vi "Login.vi"() -> ()   [LabVIEW 2018]
doc: "SubVI criada para realizar login de usuários"
uses:
  controls/Table.ctl
  controls/DataIn.ctl
  MatchDataClasses/MatchData/MatchData.lvclass
  controls/Tabuleiro.ctl
  controls/GameOption.ctl
  controls/Login - States.ctl
  controls/LoginStatus.ctl
  <vilib>/Utility/file.llb/Read Delimited Spreadsheet (string).vi
  <vilib>/Utility/file.llb/Write Delimited Spreadsheet (string).vi
panel:
  out "DataOut":T1={"Quem Joga"="", "Tabuleiro"={"(0,0)"="", "(1,0)"="", "(0,1)"="", "(1,1)"="", "(2,0)"="", "(1,2)"="", "(2,2)"="", "(0,2)"="", "(2,1) "=""}, "GameOption"=enum."Multiplayer local", "Turno"=FALSE, "Player"="", "Player 1"="", "Player 2"="", "Dificuldade"=enum."Easy", "Table"=[], "Row"=0, "Aceitar Convite"=FALSE, "Inviter line"=0, "diretório"=path "", "Logout - panel close"=FALSE, "StartGame"=FALSE, "MatchData.lvclass"=refnum, "GameMode"=enum."Single Easy"}
  in  "logout":bool
  out "Table":T4
  in  "Login":bool
  in  "User Name":string
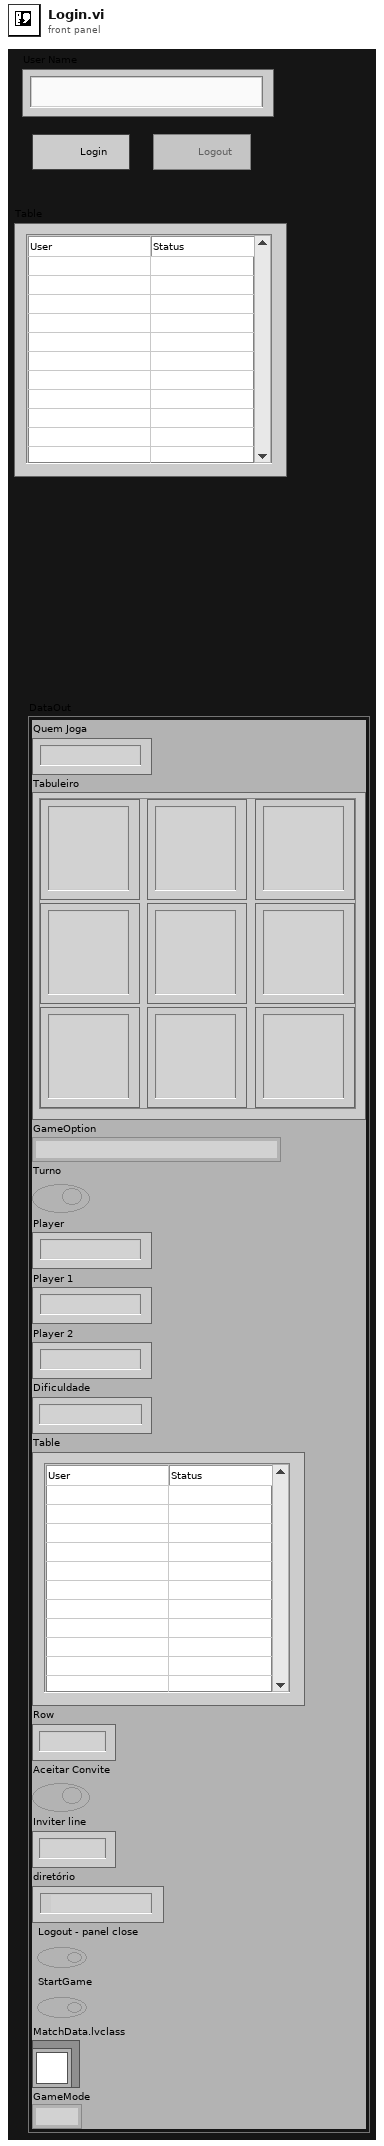
[diagram p1: front panel]
types:
  T1 = typedef "DataIn.ctl" = cluster{"Quem Joga":string, "Tabuleiro":T2, "GameOption":T3, "Turno":bool, "Player":string, "Player 1":string, "Player 2":string, "Dificuldade":enum16{"Easy", "Medium", "Hard"}, "Table":T4, "Row":u32, "Aceitar Convite":bool, "Inviter line":u32, "diretório":path, "Logout - panel close":bool, "StartGame":bool, "MatchData.lvclass":refnum<class "MatchData.lvclass">, "GameMode":enum16{"Single Easy", "Single Medium", "Single Hard", "Local", "Remote"}}
  T2 = typedef "Tabuleiro.ctl" = cluster{"(0,0)":string, "(1,0)":string, "(0,1)":string, "(1,1)":string, "(2,0)":string, "(1,2)":string, "(2,2)":string, "(0,2)":string, "(2,1) ":string}
  T3 = typedef "GameOption.ctl" = enum16{"Single Player", "Multiplayer local", "Multiplayer remoto", "Wait for Event", "Initialize", "Stop"}
  T4 = typedef "Table.ctl" = string[][]
  T5 = typedef "Login - States.ctl" = enum16{"Login - Initialize", "Login - Wait for Event", "Login", "Logout", "Table Refresh", "Invitation"}
  T6 = enum8{"Enabled", "Disabled", "Disabled and Grayed Out"}
  T7 = typedef "LoginStatus.ctl" = enum16{"File - Login", "File - Logout", "File - TableRefresh"}
  T8 = typedef "LVRowAndColumnTypeDef.ctl" = cluster{"Row":i32, "Column":i32}
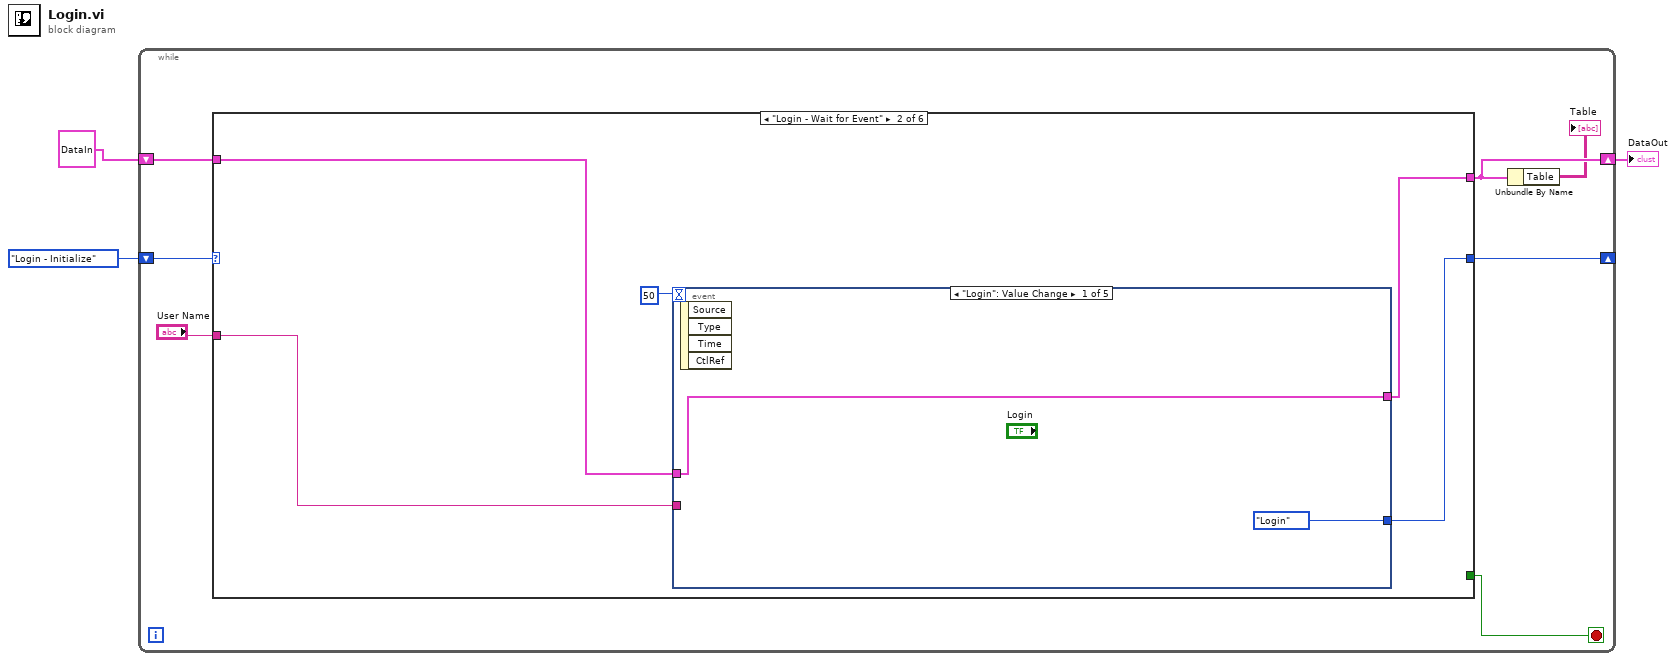
[diagram p0: block diagram]
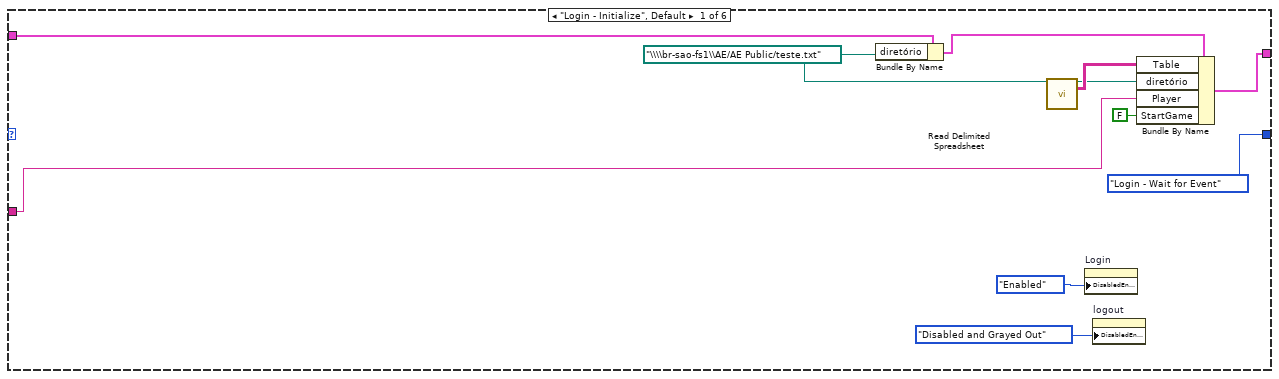
[diagram p2: hidden frame]
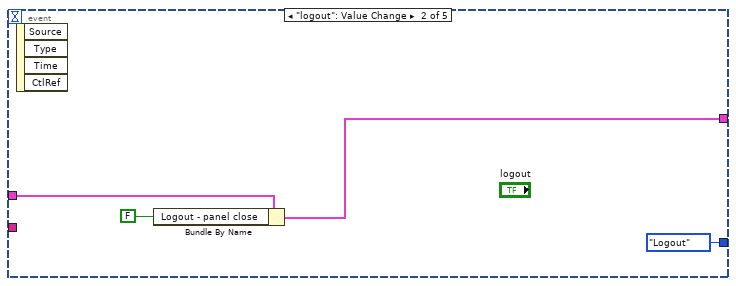
[diagram p3: hidden frame]
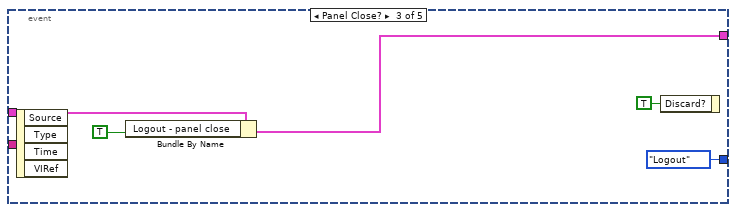
[diagram p4: hidden frame]
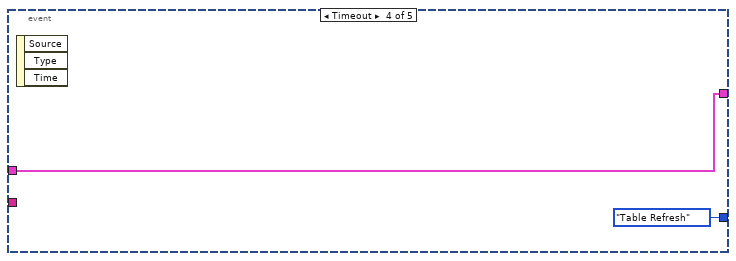
[diagram p5: hidden frame]
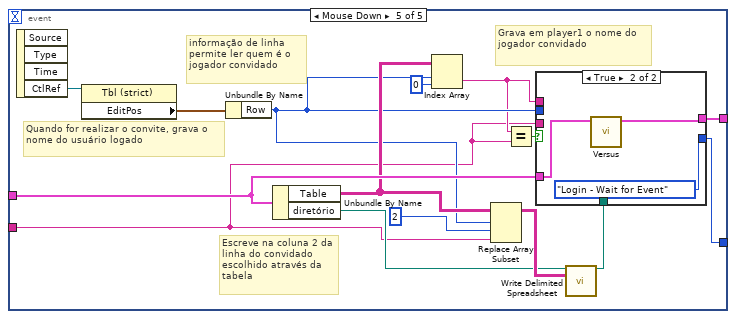
[diagram p6: hidden frame]
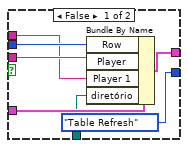
[diagram p7: hidden frame]
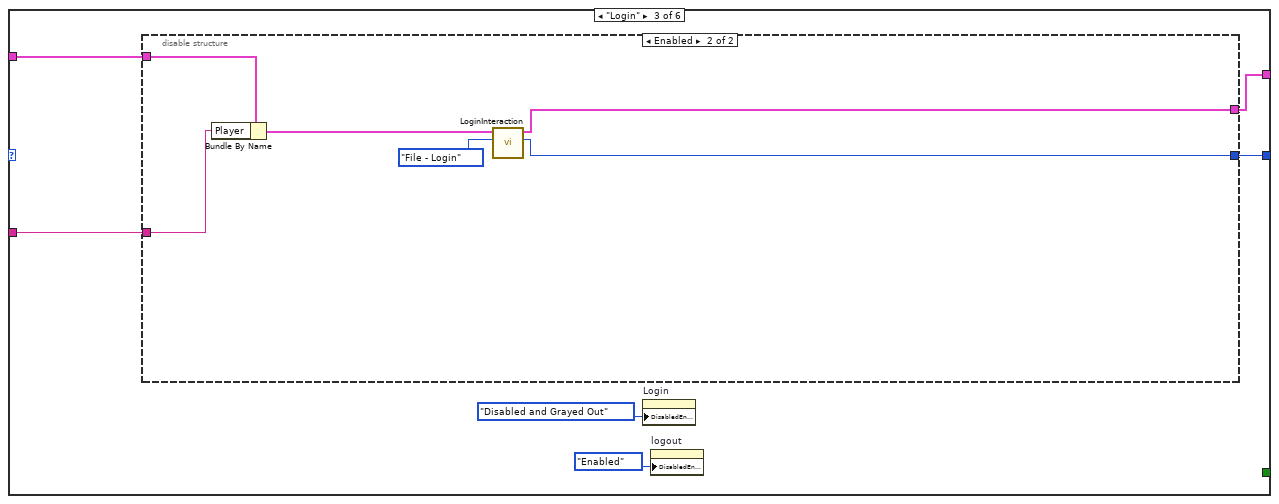
[diagram p8: hidden frame]
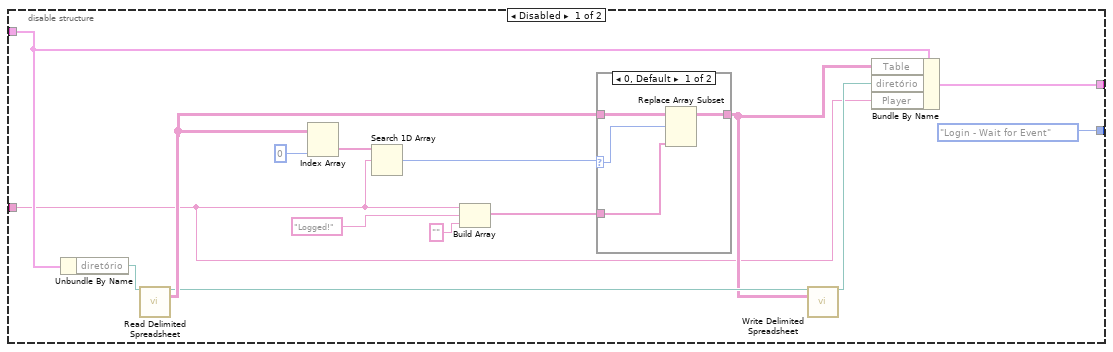
[diagram p9: hidden frame]
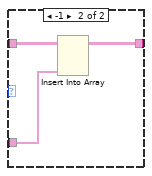
[diagram p10: hidden frame]
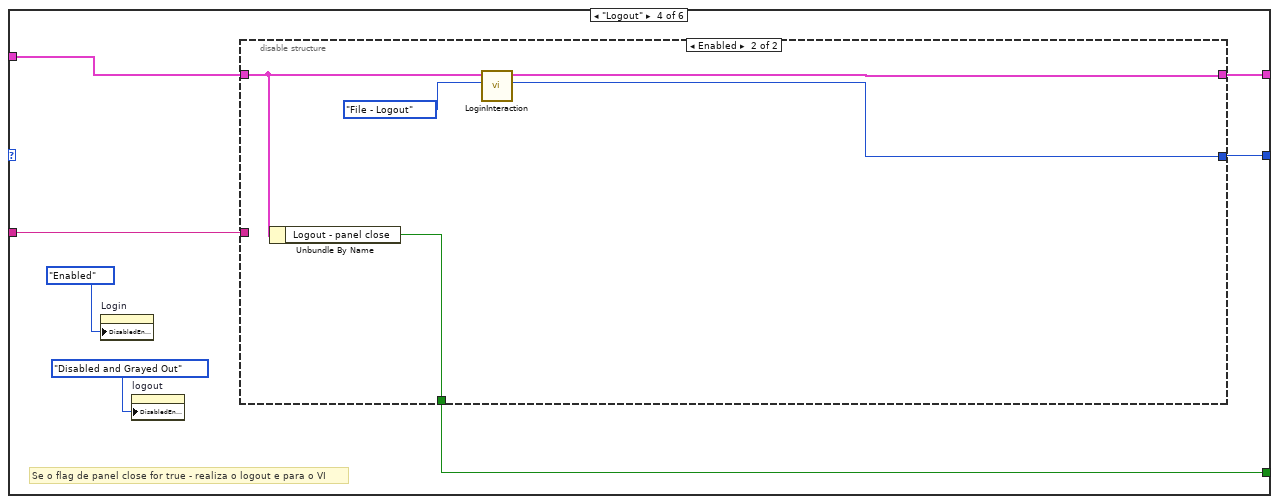
[diagram p11: hidden frame]
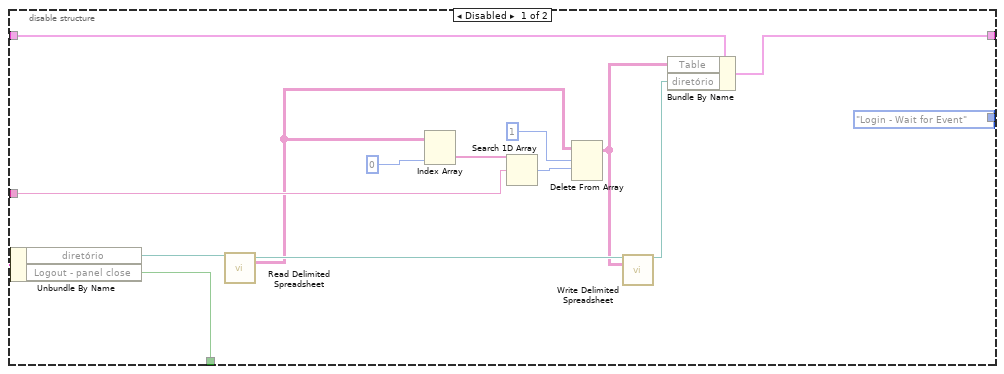
[diagram p12: hidden frame]
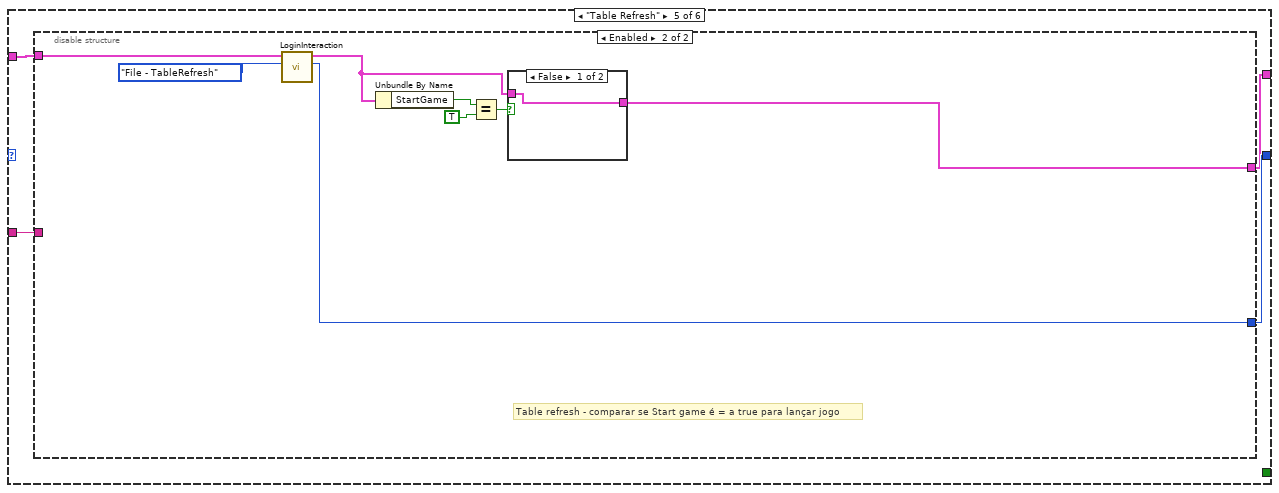
[diagram p13: hidden frame]
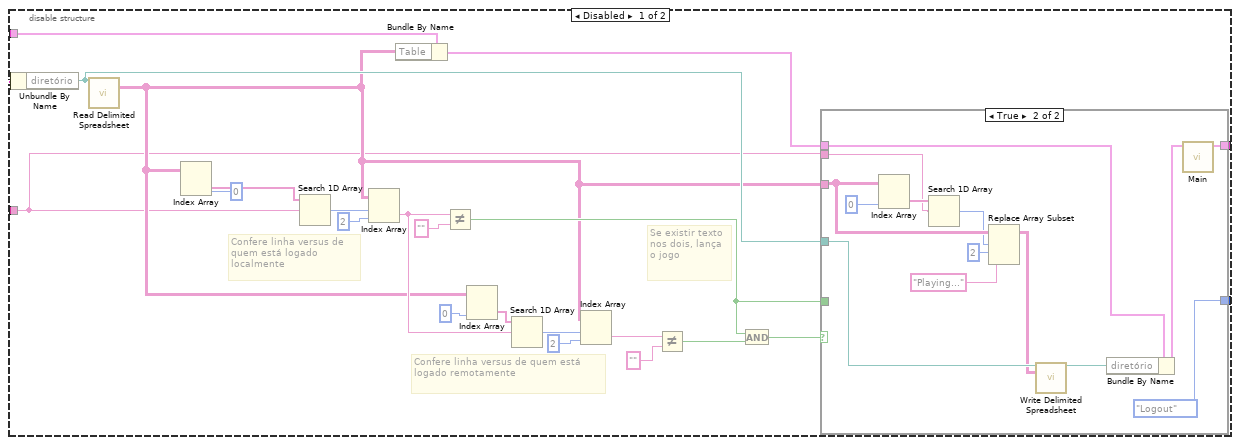
[diagram p14: hidden frame]
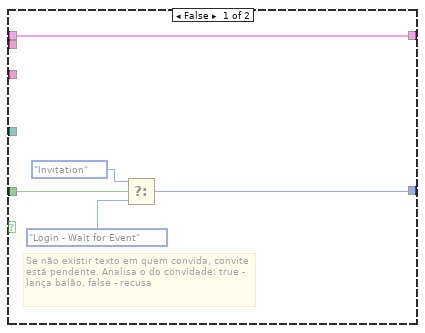
[diagram p15: hidden frame]
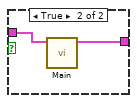
[diagram p16: hidden frame]
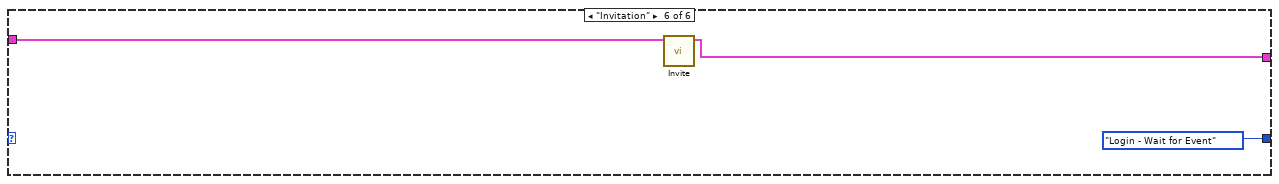
[diagram p17: hidden frame]
diagram:
  n1 = while {
    shift-right: [w9] -> _
    shift-left: Login_-_States."Login - Initialize" -> [w10]
    shift-right: [w5] -> w1
    shift-left: T1 {"Quem Joga"="", "Tabuleiro"={"(0,0)"="", "(1,0)"="", "(0,1)"="", "(1,1)"="", "(2,0)"="", "(1,2)"="", "(2,2)"="", "(0,2)"="", "(2,1) "=""}, "GameOption"=enum."Multiplayer local", "Turno"=FALSE, "Player"="", "Player 1"="", "Player 2"="", "Dificuldade"=enum."Easy", "Table"=[], "Row"=0, "Aceitar Convite"=FALSE, "Inviter line"=0, "diretório"=path "", "Logout - panel close"=FALSE, "StartGame"=FALSE, "MatchData.lvclass"=refnum, "GameMode"=enum."Single Easy"} ("DataIn") -> [w8]
    stop <- w6 stop-if-true
    n2 = case shown="\"Login - Wait for Event\"" w10 {
      tunnel: [Login_-_States."Login - Wait for Event" w26 w70 w104 w128 Login_-_States."Login - Wait for Event"] -> w9
      tunnel: w8 -> [w16 w23 w66 w99 w126 w182]
      tunnel: "User Name" -> [w12 w24 w65 w105 w125 _]
      tunnel: [_ _ _ w100 _ _] -> w6
      tunnel: [w18 w22 w67 w101 w127 w181] -> w5
      frame "Login - Initialize", Default {
        w14 = path "\\\\br-sao-fs1\\AE/AE Public/teste.txt" ("file path (use dialog)")
        n3 = Bundle By Name(cluster=w16, "diretório"=w14) -> (w15:T1)
        n4 = call-poly <vilib>:"Read Delimited Spreadsheet.vi"("file path (dialog if empty)"=w14) -> ("new file path (Not A Path if cancelled)"=w13:path, "all rows"=w17:string[][])  [unwired: 9 in, 4 out]
        n5 = property on="Login" class="Bool"("DisabledEnum"=T6."Enabled" ("Disabled")) -> ()  [unwired: 2 in, 2 out]
        n6 = property on="logout" class="Bool"("DisabledEnum"=T6."Disabled and Grayed Out" ("Disabled")) -> ()  [unwired: 2 in, 2 out]
        n7 = Bundle By Name(cluster=w15, "Table"=w17, "diretório"=w13, "Player"=w12, "StartGame"=FALSE) -> (w18:T1)
      }
      frame "Login - Wait for Event" {
        n8 = event shown="[0] \"Login\": Value Change" {
          selector: _ -> [_ _ _ _ _]
          dyn-events: _ -> [_ _ _ _ _]
          timeout: 50 -> [_ _ _ _ _]
          tunnel: [Login_-_States."Login" Login_-_States."Logout" Login_-_States."Logout" Login_-_States."Table Refresh" w40] -> w26
          tunnel: w23 -> [w27 w31 w35 w38 w51]
          tunnel: [w27 w30 w34 w38 w52] -> w22
          tunnel: w24 -> [_ _ _ _ w42]
          event "Login": Value Change {
            n9 = event-data() -> ()  [unwired: 1 in, 4 out]
          }
          event "logout": Value Change {
            n10 = event-data() -> ()  [unwired: 1 in, 4 out]
            n11 = Bundle By Name(cluster=w31, "Logout - panel close"=FALSE) -> (w30:T1)
          }
          event Panel Close? {
            n12 = event-data() -> ()  [unwired: 1 in, 4 out]
            n13 = Bundle By Name(cluster=w35, "Logout - panel close"=TRUE) -> (w34:T1)
            n14 = event-data("Discard?"=TRUE) -> ()  [unwired: 1 in, 1 out]
          }
          event Timeout {
            n15 = event-data() -> ()  [unwired: 1 in, 3 out]
          }
          event Mouse Down {
            # "Grava em player1 o nome do  jogador convidado"
            # "Escreve na coluna 2 da linha do convidado escolhido através da tabela"
            # "Quando for realizar o convite, grava o nome do usuário logado"
            # "informação de linha permite ler quem é o jogador convidado"
            n16 = event-data() -> ("CtlRef"=w54:refnum<vi>)  [unwired: 1 in, 3 out]
            n17 = property class="Tbl (strict)"(reference=w54) -> ("EditPos"=w53:T8)  [unwired: 1 in, 2 out]
            n18 = Unbundle By Name(w53) -> ("Row"=w47:i32)
            n19 = Unbundle By Name(w51) -> ("Table"=w48:T4, "diretório"=w45:path)
            n20 = Index Array(array=w48, index (row)=w47, index (col)=0 ("disabled index (col)")) -> (element=w43:string)
            n21 = Replace Array Subset(array=w48, new element=w42, index (row)=w47, index (col)=2 ("disabled index (col)")) -> (w50:T4)
            n22 = Equal?(x=w43, y=w42) -> (x = y?=w41:bool)
            n23 = call-poly <vilib>:"Write Delimited Spreadsheet.vi"("file path (dialog if empty)"=w45, "2D data"=w50) -> ("new file path (Not A Path if cancelled)"=w44:path)  [unwired: 12 in, 1 out]
            n24 = case shown="True" w41 {
              tunnel: [w61 w63] -> w52
              tunnel: w51 -> [w60 w62]
              tunnel: w42 -> [w59 _]
              tunnel: w47 -> [w58 _]
              tunnel: w43 -> [w57 _]
              tunnel: w44 -> [w56 _]
              tunnel: [Login_-_States."Table Refresh" Login_-_States."Login - Wait for Event"] -> w40
              frame False {
                n25 = Bundle By Name(cluster=w60, "Row"=w58, "Player"=w59, "Player 1"=w57, "diretório"=w56) -> (w61:T1)
              }
              frame True {
                n26 = call "Versus.vi"("DataIn"=w62) -> ("DataOut"=w63:T1)  [unwired: 10 in]
              }
            }
          }
        }
      }
      frame "Login" {
        n27 = disable-structure shown="Enabled" {
          disable-tunnel: [Login_-_States."Login - Wait for Event" w93] -> w70
          disable-tunnel: [w76 w94] -> w67
          disable-tunnel: w66 -> [w74 w97]
          disable-tunnel: w65 -> [w71 w95]
          frame Disabled {
            n28 = Unbundle By Name(w74) -> ("diretório"=w73:path)
            n29 = call-poly <vilib>:"Read Delimited Spreadsheet.vi"("file path (dialog if empty)"=w73) -> ("new file path (Not A Path if cancelled)"=w84:path, "all rows"=w85:string[][])  [unwired: 9 in, 4 out]
            n30 = Index Array(array=w85, index (col)=0 ("index (row)")) -> (element=w79:string[])  [unwired: 1 in]
            n31 = Search 1D Array(1D array=w79, element=w71) -> (index of element=w83:i32)  [unwired: 1 in]
            n32 = Build Array(w71, "Logged!" ("input 2"), "" ("element")) -> (w81:string[])
            n33 = case shown="0, Default" w83 {
              selector: w83 -> [w86 _]
              tunnel: w85 -> [w89 w92]
              tunnel: w81 -> [w88 w91]
              tunnel: [w87 w90] -> w75
              frame 0, Default {
                n34 = Replace Array Subset(array=w89, new element=w88, index (row)=w86) -> (w87:string[][])  [unwired: 1 in]
              }
              frame -1 {
                n35 = Insert Into Array(array=w92, new element=w91) -> (w90:string[][])  [unwired: 2 in]
              }
            }
            n36 = call-poly <vilib>:"Write Delimited Spreadsheet.vi"("file path (dialog if empty)"=w84, "2D data"=w75) -> ("new file path (Not A Path if cancelled)"=w72:path)  [unwired: 12 in, 1 out]
            n37 = Bundle By Name(cluster=w74, "Table"=w75, "diretório"=w72, "Player"=w71) -> (w76:T1)
          }
          frame Enabled {
            n38 = Bundle By Name(cluster=w97, "Player"=w95) -> (w96:T1)
            n39 = call "LoginInteraction.vi"("LoginStatus"=LoginStatus."File - Login", "DataIn"=w96) -> ("NextState"=w93:T5, "DataOut"=w94:T1)  [unwired: 8 in]
          }
        }
        n40 = property on="Login" class="Bool"("DisabledEnum"=T6."Disabled and Grayed Out" ("Disabled")) -> ()  [unwired: 2 in, 2 out]
        n41 = property on="logout" class="Bool"("DisabledEnum"=T6."Enabled" ("Disabled")) -> ()  [unwired: 2 in, 2 out]
      }
      frame "Logout" {
        # "Se o flag de panel close for true - realiza o logout e para o VI"
        n42 = property on="Login" class="Bool"("DisabledEnum"=T6."Enabled" ("Disabled")) -> ()  [unwired: 2 in, 2 out]
        n43 = property on="logout" class="Bool"("DisabledEnum"=T6."Disabled and Grayed Out" ("Disabled")) -> ()  [unwired: 2 in, 2 out]
        n44 = disable-structure shown="Enabled" {
          disable-tunnel: w105 -> [w116 _]
          disable-tunnel: [Login_-_States."Login - Wait for Event" w122] -> w104
          disable-tunnel: [w111 w123] -> w101
          disable-tunnel: [w107 w120] -> w100
          disable-tunnel: w99 -> [w106 w121]
          frame Disabled {
            n45 = Unbundle By Name(w106) -> ("diretório"=w109:path, "Logout - panel close"=w107:bool)
            n46 = call-poly <vilib>:"Read Delimited Spreadsheet.vi"("file path (dialog if empty)"=w109) -> ("new file path (Not A Path if cancelled)"=w119:path, "all rows"=w114:string[][])  [unwired: 9 in, 4 out]
            n47 = Index Array(array=w114, index (col)=0 ("disabled index (col)")) -> (element=w118:string[])  [unwired: 1 in]
            n48 = Search 1D Array(1D array=w118, element=w116) -> (index of element=w113:i32)  [unwired: 1 in]
            n49 = Delete From Array(array=w114, length=1, index (row)=w113) -> (array with subset deleted=w110:string[][])  [unwired: 1 in, 1 out]
            n50 = call-poly <vilib>:"Write Delimited Spreadsheet.vi"("file path (dialog if empty)"=w119, "2D data"=w110) -> ("new file path (Not A Path if cancelled)"=w108:path)  [unwired: 12 in, 1 out]
            n51 = Bundle By Name(cluster=w106, "Table"=w110, "diretório"=w108) -> (w111:T1)
          }
          frame Enabled {
            n52 = Unbundle By Name(w121) -> ("Logout - panel close"=w120:bool)
            n53 = call "LoginInteraction.vi"("LoginStatus"=LoginStatus."File - Logout", "DataIn"=w121) -> ("NextState"=w122:T5, "DataOut"=w123:T1)  [unwired: 8 in]
          }
        }
      }
      frame "Table Refresh" {
        n54 = disable-structure shown="Enabled" {
          disable-tunnel: [w135 w170] -> w128
          disable-tunnel: [w133 w171] -> w127
          disable-tunnel: w126 -> [w132 w177]
          disable-tunnel: w125 -> [w129 _]
          frame Disabled {
            # "Se existir texto nos dois, lança o jogo"
            # "Confere linha versus de quem está logado remotamente"
            # "Confere linha versus de quem está logado localmente"
            n55 = Unbundle By Name(w132) -> ("diretório"=w131:path)
            n56 = call-poly <vilib>:"Read Delimited Spreadsheet.vi"("file path (dialog if empty)"=w131) -> ("all rows"=w130:string[][])  [unwired: 9 in, 5 out]
            n57 = Index Array(array=w130, index (col)=0 ("disabled index (col)")) -> (element=w149:string[])  [unwired: 1 in]
            n58 = Search 1D Array(1D array=w149, element=w129) -> (index of element=w146:i32)  [unwired: 1 in]
            n59 = Index Array(array=w130, index (row)=w146, index (col)=2) -> (element=w140:string)
            n60 = Bundle By Name(cluster=w132, "Table"=w130) -> (w134:T1)
            n61 = Not Equal?(x=w140, y="") -> (x != y?=w136:bool)
            n62 = Index Array(array=w130, index (col)=0 ("disabled index (col)")) -> (element=w142:string[])  [unwired: 1 in]
            n63 = Search 1D Array(1D array=w142, element=w140) -> (index of element=w145:i32)  [unwired: 1 in]
            n64 = Index Array(array=w130, index (row)=w145, index (col)=2) -> (element=w139:string)
            n65 = Not Equal?(x=w139, y="") -> (x != y?=w138:bool)
            n66 = And(x=w136, y=w138) -> (x .and. y?=w137:bool)
            n67 = case shown="True" w137 {
              tunnel: w136 -> [w155 _]
              tunnel: [w152 Login_-_States."Logout"] -> w135
              tunnel: w134 -> [w151 w159]
              tunnel: [w151 w157] -> w133
              tunnel: w131 -> [_ w168]
              tunnel: w130 -> [_ w164]
              tunnel: w129 -> [_ w165]
              frame False {
                # "Se não existir texto em quem convida, convite está pendente. Analisa o do convidade: true - lança balão, false - recusa"
                n68 = Select(t=Login_-_States."Invitation" ("f"), s=w155, f=Login_-_States."Login - Wait for Event") -> (s? t:f=w152:T5)
              }
              frame True {
                n69 = Index Array(array=w164, index (col)=0 ("index (row)")) -> (element=w166:string[])  [unwired: 1 in]
                n70 = Search 1D Array(1D array=w166, element=w165) -> (index of element=w162:i32)  [unwired: 1 in]
                n71 = Replace Array Subset(array=w164, new element="Playing..." ("new element/subarray"), index (row)=w162, index (col)=2 ("disabled index (col)")) -> (w160:string[][])
                n72 = call-poly <vilib>:"Write Delimited Spreadsheet.vi"("file path (dialog if empty)"=w168, "2D data"=w160) -> ("new file path (Not A Path if cancelled)"=w158:path)  [unwired: 12 in, 1 out]
                n73 = Bundle By Name(cluster=w159, "diretório"=w158) -> (w156:T1)
                n74 = call "Main.vi"("DataIn"=w156) -> ("DataOut"=w157:T1)  [unwired: 10 in]
              }
            }
          }
          frame Enabled {
            # "Table refresh - comparar se Start game é = a true para lançar jogo"
            n75 = call "LoginInteraction.vi"("LoginStatus"=LoginStatus."File - TableRefresh", "DataIn"=w177) -> ("NextState"=w170:T5, "DataOut"=w172:T1)  [unwired: 8 in]
            n76 = Unbundle By Name(w172) -> ("StartGame"=w175:bool)
            n77 = Equal?(x=w175, y=TRUE) -> (x = y?=w173:bool)
            n78 = case shown="False" w173 {
              tunnel: w172 -> [w178 w180]
              tunnel: [w178 w179] -> w171
              frame False {
              }
              frame True {
                n79 = call "Main.vi"("DataIn"=w180) -> ("DataOut"=w179:T1)  [unwired: 10 in]
              }
            }
          }
        }
      }
      frame "Invitation" {
        n80 = call "Invite.vi"("DataIn"=w182) -> ("DataOut"=w181:T1)  [unwired: 9 in]
      }
    }
    n81 = Unbundle By Name(w5) -> ("Table"=→"Table":T4)
  }
  "DataOut" <- w1
